vi "Create Tree.vi"(7 "Parent ID (empty)":string, 8 "Error In":errorcluster, 9 "Attributes Dictionary":variant, 10 "Name":string, 11 "Tree Manager":T1) -> (0 "Error Out":errorcluster, 3 "Tree Manager":T1, 5 "Unique ID":string)   [LabVIEW 2016, in "Tree Manager.lvclass"]
doc: "Create a new Tree in the Tree Manager and assign to it a Unique ID. Use this Unique ID to interact with this tree.\n\nThe Data input can contain a set of variant attributes that will be used as the Tree attributes.\n\nYou can provide the optional Parent ID input if you want to create the Child Tree directly under already existing Parent.\n\n<b>WARNING</b> The name Attribute is reserved by the Tree API. Do not use that name for your Trees."
uses:
  Tree Manager.lvclass
  Typedefs/Session Handle.ctl
  Tree Manager.lvclass/Tree Manager.ctl
  <vilib>/Utility/error.llb/Error Cluster From Error Code.vi
  <vilib>/ErrorRing/Error Ring.xnode
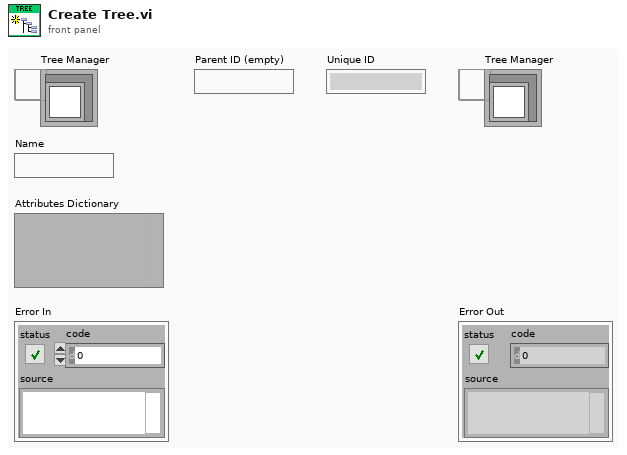
[diagram p1: front panel]
types:
  T1 = typedef "Tree Manager.lvclass/Session Handle.ctl" = refnum<data-value>
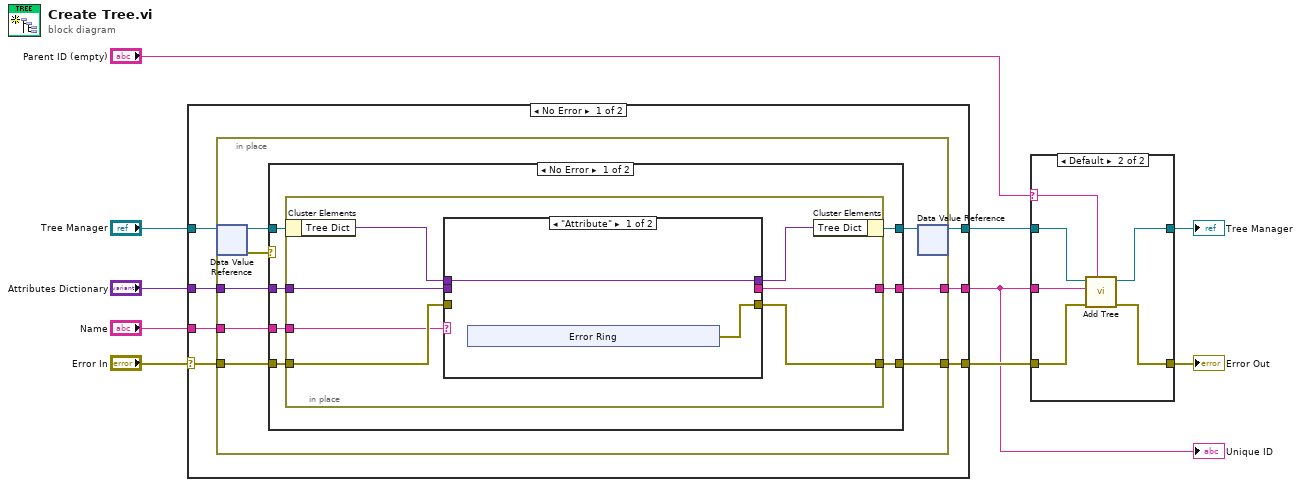
[diagram p0: block diagram]
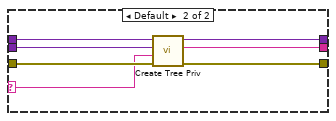
[diagram p3: hidden frame]
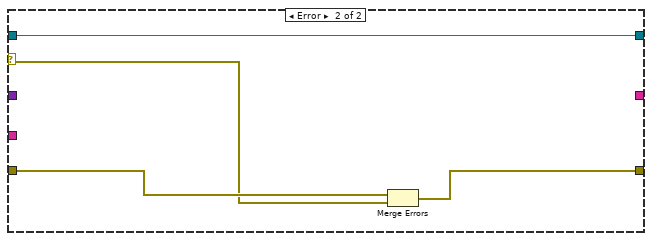
[diagram p4: hidden frame]
diagram:
  n1 = case shown="No Error" "Error In" {
    selector: "Error In" -> [w15 w58]
    tunnel: "Tree Manager" -> [w17 w59]
    tunnel: [w16 w59] -> w7
    tunnel: [w14 w58] -> w8
    tunnel: "Attributes Dictionary" -> [w13 _]
    tunnel: "Name" -> [w12 _]
    tunnel: [w11 _] -> w5
    frame No Error {
      n2 = in-place {
        in-place-border: w15 -> [w21]
        in-place-border: [w24] -> w14
        in-place-border: w13 -> [w20]
        in-place-border: w12 -> [w19]
        in-place-border: [w18] -> w11
        n3 = in-place-dvr #1(w17) -> (w25:refnum<class "Tree Manager.lvclass">, w22:errorcluster)
        n4 = case shown="No Error" w22 {
          selector: w22 -> [_ w56]
          tunnel: w25 -> [w32 w54]
          tunnel: [w31 w55] -> w24
          tunnel: [w30 w54] -> w23
          tunnel: w21 -> [w29 w57]
          tunnel: w20 -> [w28 _]
          tunnel: w19 -> [w27 _]
          tunnel: [w26 _] -> w18
          frame No Error {
            n5 = in-place {
              in-place-border: [w36] -> w31
              in-place-border: w29 -> [w37]
              in-place-border: w28 -> [w35]
              in-place-border: w27 -> [w33]
              in-place-border: [w34] -> w26
              n6 = in-place-cluster #2(w32) -> ("Tree Dict"=w39:variant)
              n7 = case shown="\"Attribute\"" w33 {
                selector: w33 -> [_ w47]
                tunnel: w39 -> [w41 w53]
                tunnel: [w41 w52] -> w38
                tunnel: w37 -> [_ w51]
                tunnel: [w40 w50] -> w36
                tunnel: w35 -> [_ w49]
                tunnel: [_ w48] -> w34
                frame "Attribute" {
                  n8 = xnode "Error Ring"() -> ("error out"=w40:errorcluster)
                }
                frame Default {
                  n9 = call "Create Tree Priv.vi"("Error In"=w51, "Name"=w47, "Data"=w49, "Tree Dictionary In"=w53) -> ("Error Out"=w50:errorcluster, "Unique ID"=w48:string, "Tree Dictionary Out"=w52:variant)  [unwired: 5 in]
                }
              }
              n10 = in-place-cluster #2("Tree Dict"=w38) -> (w30:refnum<class "Tree Manager.lvclass">)
            }
          }
          frame Error {
            n11 = Merge Errors(w57, w56) -> (w55:errorcluster)
          }
        }
        n12 = in-place-dvr #1(w23) -> (w16:T1)  [unwired: 1 out]
      }
    }
    frame Error {
    }
  }
  "Unique ID" <- w5
  n13 = case shown="Default" "Parent ID (empty)" {
    selector: "Parent ID (empty)" -> [_ w63]
    tunnel: w8 -> [w60 w67]
    tunnel: [w60 w66] -> w1
    tunnel: w7 -> [w61 w65]
    tunnel: [w61 w64] -> w2
    tunnel: w5 -> [_ w62]
    frame "" {
    }
    frame Default {
      n14 = call "Add Tree.vi"("Parent ID"=w63, "Error In"=w67, "Child ID"=w62, "Tree Manager"=w65) -> ("Error Out"=w66:errorcluster, "Tree Manager"=w64:T1)  [unwired: 6 in]
    }
  }
  "Tree Manager" <- w2
  "Error Out" <- w1
